vi "Integer2ByteArray.vi"(1 "Integer":u32) -> (0 "Byte Array":u8[](array[numeric]))   [LabVIEW 2016, in "Brooks MFC.lvclass"]
uses:
  Brooks MFC.lvclass
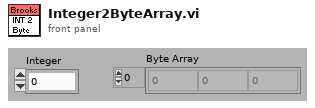
[diagram p1: front panel]
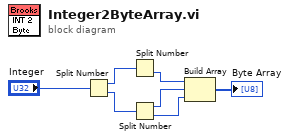
[diagram p0: block diagram]
diagram:
  n1 = Split Number(x="Integer") -> (hi(x)=w6:u16, lo(x)=w5:u16)
  n2 = Split Number(x=w6) -> (lo(x)=w4:u8)  [unwired: 1 out]
  n3 = Split Number(x=w5) -> (hi(x)=w3:u8, lo(x)=w2:u8)
  n4 = Build Array(w4, w3, w2) -> (→"Byte Array":u8[])
